vi "DiffDrvAccelLimit_Calculate.vi"(6 "RightVoltage":dbl, 8 "LeftVoltage":dbl, 9 "RightVelocity":dbl, 10 "LeftVelocity":dbl, 11 "inDiffDriveAccelLimit":T1) -> (0 "Error":bool, 2 "NewRightVoltage":dbl, 3 "NewLeftVoltage":dbl)   [LabVIEW 2019, in "Trajectory_Library.lvlib"]
doc: "Calculate the accelerationlimited differential drive output voltages \nInputs:\n - DiffDriveAccelLimit -- Data cluster\n\nOutputs:\n - Error -- If TRUE, an error occured."
uses:
  Trajectory_Library.lvlib
  DIFF_DRIVE_ACCEL_LIMIT.ctl
  LINEAR_SYSTEM.ctl
  <vilib>/Analysis/Matrix/Datatypes/RealMatrix.ctl
  <vilib>/Analysis/baseanly.llb/Real A x B.vi
  MatBuilder_Create.vi
  <vilib>/Analysis/Matrix/Numeric/Add/Add - RM,RM.vi
  <vilib>/Analysis/7linalg.llb/Solve Linear Equations (multiple right hand).vi
  <vilib>/Analysis/Matrix/Numeric/Subtract/Subtract - RM,RM.vi
  <vilib>/Analysis/NI_AALBase.lvlib
  <vilib>/Analysis/Matrix/NI_Matrix.lvlib
  <vilib>/Analysis/NI_AALPro.lvlib
panel:
  # "NOTE --- PERHAPS THE SYSTEM SHOULD NOT BE PART OF THE CLUSTER"
  # "<States,States>"
  # "<States,Inputs>"
  # "<Outputs,States>"
  # "<Outputs,Inputs>"
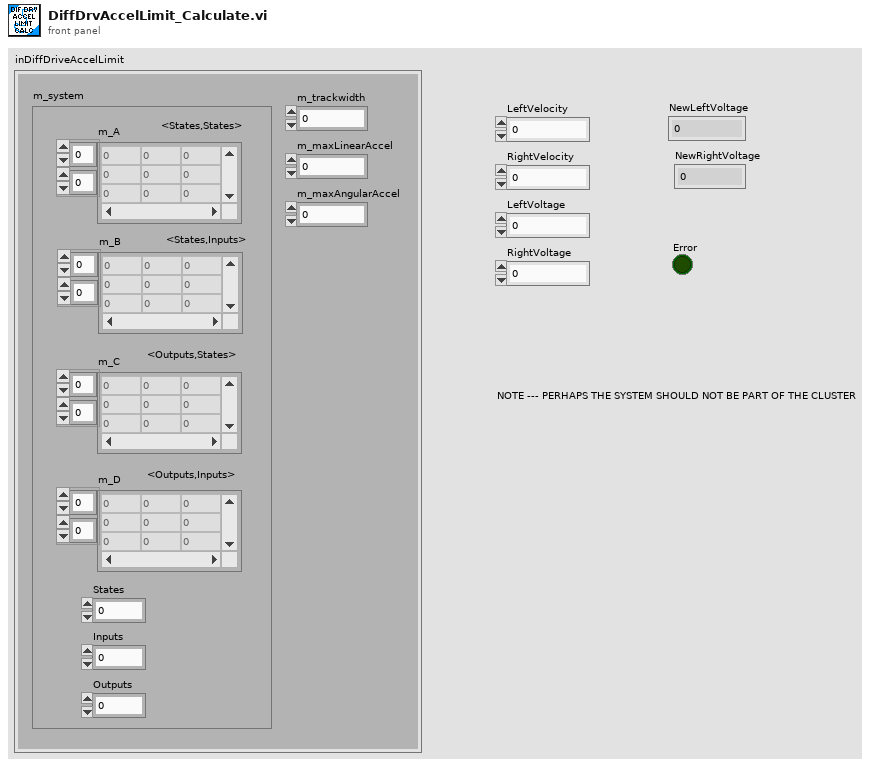
[diagram p1: front panel]
types:
  T1 = typedef "Trajectory_Library.lvlib/DIFF_DRIVE_ACCEL_LIMIT.ctl" = cluster{"m_system":T2, "m_trackwidth":dbl, "m_maxLinearAccel":dbl, "m_maxAngularAccel":dbl}
  T2 = typedef "Trajectory_Library.lvlib/LINEAR_SYSTEM.ctl" = cluster{"m_A":T3, "m_B":T3, "m_C":T3, "m_D":T3, "States":i32, "Inputs":i32, "Outputs":i32}
  T3 = typedef "NI_Matrix.lvlib/RealMatrix.ctl" = dbl[][]
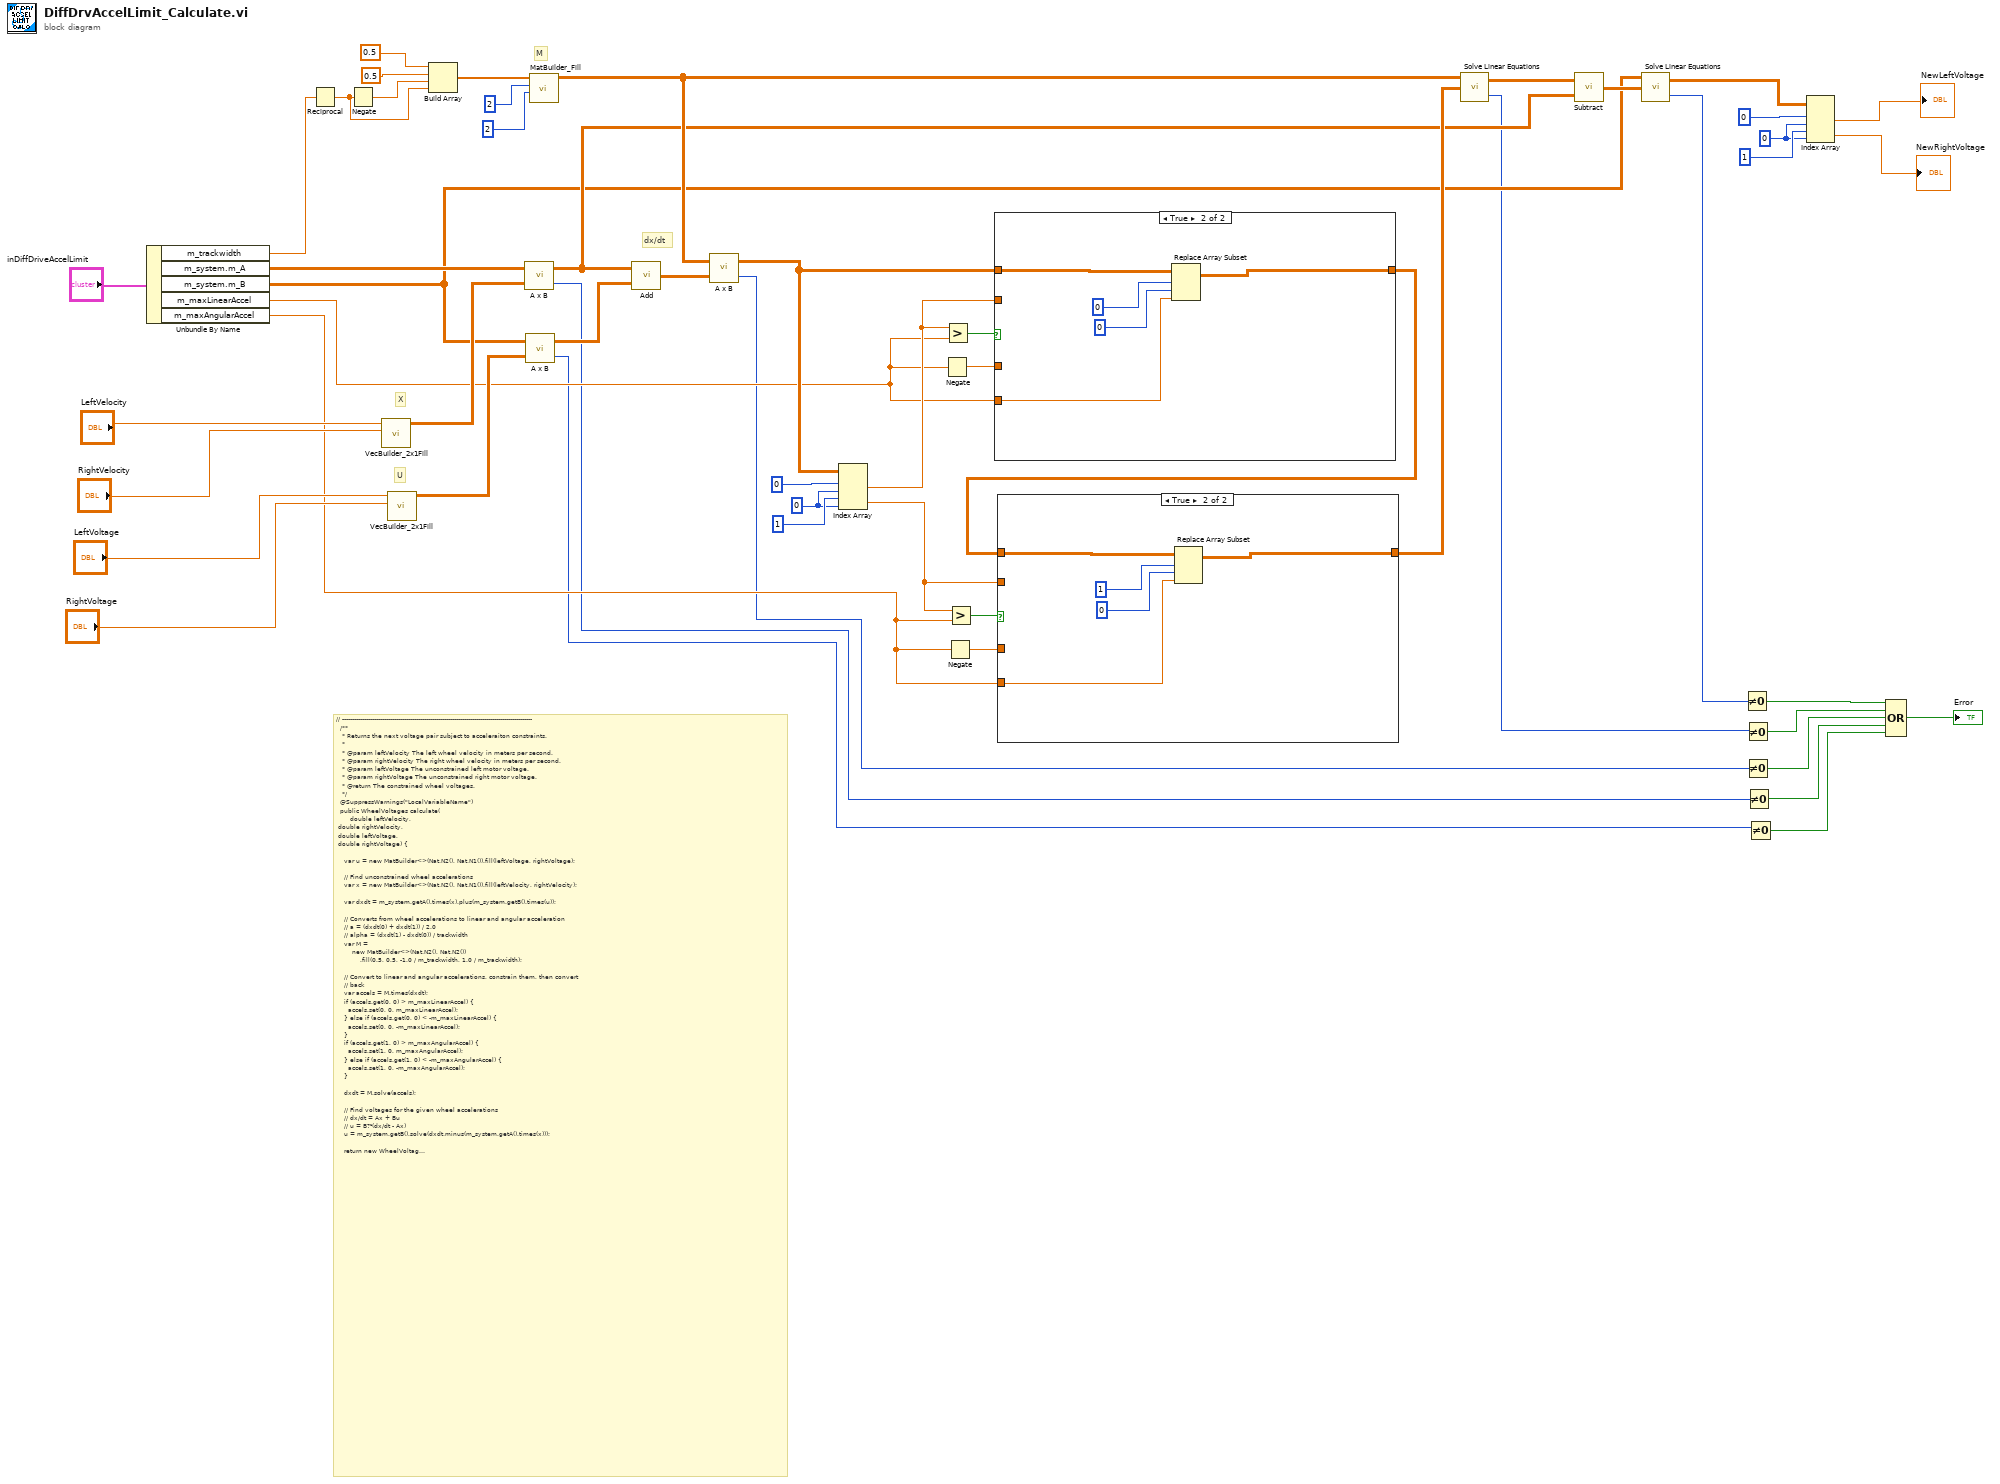
[diagram p0: block diagram]
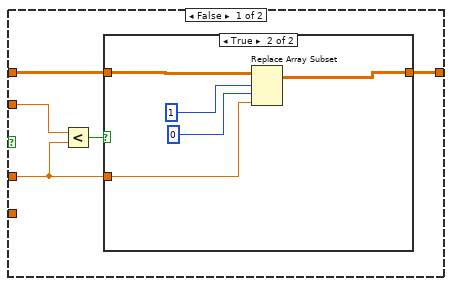
[diagram p2: hidden frame]
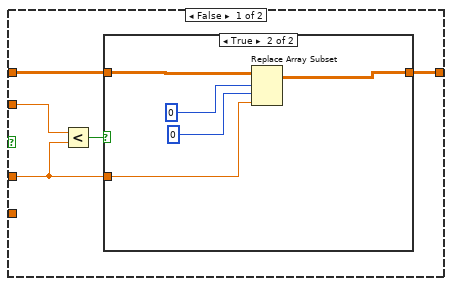
[diagram p4: hidden frame]
diagram:
  w21 = 0 ("index (col)")
  w35 = 0 ("index (col)")
  # "dx/dt"
  # "M"
  # "U"
  # "X"
  # "// -----------------------------------------------------------------------------------------------\n  /**\n   * Returns the next voltage pair subject to acceleraiton constraints.\n   *\n   * @param leftVelocity The left wheel velocity in meters per second.\n   * @param rightVelocity The right wheel velocity in meters per second.\n   * @param leftVoltage The unconstrained left motor voltage.\n   * @param rightVoltage The unconstrained right motor voltage.\n   * @return The constrained wheel voltages.\n   */\n  @SuppressWarnings(\"LocalVariableName\")\n  public WheelVoltages calculate(\n      \tdouble leftVelocity, \n\tdouble rightVelocity, \n\tdouble leftVoltage, \n\tdouble rightVoltage) {\n\n    var u = new MatBuilder<>(Nat.N2(), Nat.N1()).fill(leftVoltage, rightVoltage);\n\n    // Find unconstrained wheel accelerations\n    var x = new MatBuilder<>(Nat.N2(), Nat.N1()).fill(leftVelocity, rightVelocity);\n\n    var dxdt = m_system.getA().times(x).plus(m_system.getB().times(u));\n\n    // Converts from wheel accelerations to linear and angular acceleration\n    // a = (dxdt(0) + dxdt(1)) / 2.0\n    // alpha = (dxdt(1) - dxdt(0)) / trackwidth\n    var M =\n        new MatBuilder<>(Nat.N2(), Nat.N2())\n            .fill(0.5, 0.5, -1.0 / m_trackwidth, 1.0 / m_trackwidth);\n\n    // Convert to linear and angular accelerations, constrain them, then convert\n    // back\n    var accels = M.times(dxdt);\n    if (accels.get(0, 0) > m_maxLinearAccel) {\n      accels.set(0, 0, m_maxLinearAccel);\n    } else if (accels.get(0, 0) < -m_maxLinearAccel) {\n      accels.set(0, 0, -m_maxLinearAccel);\n    }\n    if (accels.get(1, 0) > m_maxAngularAccel) {\n      accels.set(1, 0, m_maxAngularAccel);\n    } else if (accels.get(1, 0) < -m_maxAngularAccel) {\n      accels.set(1, 0, -m_maxAngularAccel);\n    }\n\n    dxdt = M.solve(accels);\n\n    // Find voltages for the given wheel accelerations\n    // dx/dt = Ax + Bu\n    // u = B?¹(dx/dt - Ax)\n    u = m_system.getB().solve(dxdt.minus(m_system.getA().times(x)));\n\n    return new WheelVoltages(u.get(0, 0), u.get(1, 0));\n  }"
  n1 = Unbundle By Name("inDiffDriveAccelLimit") -> ("m_trackwidth"=w1:dbl, "m_system.m_A"=w49:T3, "m_system.m_B"=w16:T3, "m_maxLinearAccel"=w27:dbl, "m_maxAngularAccel"=w17:dbl)
  n2 = Reciprocal(x=w1) -> (1/x=w39:dbl)
  n3 = Negate(x=w39) -> (-x=w40:dbl)
  n4 = call "VecBuilder_2x1Fill.vi"("R1"="RightVelocity", "R0"="LeftVelocity") -> ("output matrix"=w48:T3)  [unwired: 9 in]
  n5 = call "VecBuilder_2x1Fill.vi"("R1"="RightVoltage", "R0"="LeftVoltage") -> ("output matrix"=w47:T3)  [unwired: 9 in]
  n6 = Build Array(0.5 ("element"), 0.5 ("element"), w40, w39) -> (w45:dbl[])
  n7 = call-poly <vilib>:"A x B.vi"("B"=w48, "A"=w49) -> ("error"=w9:i32, "A x B"=w19:T3)
  n8 = call-poly <vilib>:"A x B.vi"("B"=w47, "A"=w16) -> ("error"=w8:i32, "A x B"=w46:T3)
  n9 = call "MatBuilder_Fill.vi"("Columns"=2, "Rows"=2, "Value List"=w45) -> ("output matrix"=w25:T3)  [unwired: 8 in]
  n10 = call-poly <vilib>:"Add.vi"("Real Matrix B"=w46, "Real Matrix A"=w19) -> ("A + B"=w38:T3)
  n11 = call-poly <vilib>:"A x B.vi"("B"=w38, "A"=w25) -> ("error"=w10:i32, "A x B"=w31:T3)
  n12 = Index Array(array=w31, index (row) #1=0 ("index (row)"), index (col) #1=w35, index (row) #2=1 ("index (row)"), index (col) #2=w35) -> (element #1=w33:dbl, element #2=w28:dbl)
  n13 = Negate(x=w27) -> (-x=w32:dbl)
  n14 = Greater?(x=w33, y=w27) -> (0:w34:bool)
  n15 = Negate(x=w17) -> (-x=w29:dbl)
  n16 = Greater?(x=w28, y=w17) -> (0:w30:bool)
  n17 = case shown="True" w34 {
    tunnel: w33 -> [w58 _]
    tunnel: w32 -> [w55 _]
    tunnel: w31 -> [w57 w70]
    tunnel: [w56 w66] -> w26
    tunnel: w27 -> [_ w67]
    frame False {
      n18 = Less?(x=w58, y=w55) -> (x < y?=w59:bool)
      n19 = case shown="True" w59 {
        tunnel: w57 -> [w60 w62]
        tunnel: [w60 w61] -> w56
        tunnel: w55 -> [_ w63]
        frame False {
        }
        frame True {
          n20 = Replace Array Subset(array=w62, new element=w63, index (row)=0 ("disabled index (row)"), index (col)=0 ("disabled index (col)")) -> (w61:T3)
        }
      }
    }
    frame True {
      n21 = Replace Array Subset(array=w70, new element=w67, index (row)=0 ("disabled index (row)"), index (col)=0 ("disabled index (col)")) -> (w66:T3)
    }
  }
  n22 = case shown="True" w30 {
    tunnel: w28 -> [w74 _]
    tunnel: w29 -> [w71 _]
    tunnel: w26 -> [w73 w86]
    tunnel: [w72 w82] -> w24
    tunnel: w17 -> [_ w83]
    frame False {
      n23 = Less?(x=w74, y=w71) -> (x < y?=w75:bool)
      n24 = case shown="True" w75 {
        tunnel: w73 -> [w76 w78]
        tunnel: [w76 w77] -> w72
        tunnel: w71 -> [_ w79]
        frame False {
        }
        frame True {
          n25 = Replace Array Subset(array=w78, new element=w79, index (row)=1 ("disabled index (row)"), index (col)=0 ("disabled index (col)")) -> (w77:T3)
        }
      }
    }
    frame True {
      n26 = Replace Array Subset(array=w86, new element=w83, index (row)=1 ("disabled index (row)"), index (col)=0 ("disabled index (col)")) -> (w82:T3)
    }
  }
  n27 = call-poly <vilib>:"Solve Linear Equations.vi"("Known Matrix"=w24, "Input Matrix"=w25) -> ("error"=w11:i32, "Solution Matrix"=w20:T3)  [unwired: 1 in]
  n28 = call-poly <vilib>:"Subtract.vi"("Real Matrix B"=w19, "Real Matrix A"=w20) -> ("A - B"=w18:T3)
  n29 = call-poly <vilib>:"Solve Linear Equations.vi"("Known Matrix"=w18, "Input Matrix"=w16) -> ("error"=w12:i32, "Solution Matrix"=w15:T3)  [unwired: 1 in]
  n30 = Not Equal To 0?(x=w12) -> (x != 0?=w7:bool)
  n31 = Not Equal To 0?(x=w11) -> (x != 0?=w6:bool)
  n32 = Not Equal To 0?(x=w10) -> (x != 0?=w5:bool)
  n33 = Not Equal To 0?(x=w9) -> (x != 0?=w4:bool)
  n34 = Not Equal To 0?(x=w8) -> (x != 0?=w3:bool)
  n35 = Index Array(array=w15, index (row) #1=0 ("index (row)"), index (col) #1=w21, index (row) #2=1 ("index (row)"), index (col) #2=w21) -> (element #1=→"NewLeftVoltage":dbl, element #2=→"NewRightVoltage":dbl)
  n36 = Compound Arithmetic op=OR(w7, w6, w5, w4, w3) -> (→"Error":bool)
